vi "run.create_set_end.vi"(8 "error in":errorcluster, 10 "Time Stamp (Now)":timestamp format="%<%x %.3X>T", 11 "RunCreateStaging in":refnum<class "RunCreateStaging.lvclass">) -> (0 "error out":errorcluster, 3 "RunCreateStaging out":refnum<class "RunCreateStaging.lvclass">)   [LabVIEW 2020, in "RunCreateStaging.lvclass"]
doc: "Sets the end time for the run being created."
uses:
  RunCreateStaging.lvclass
  RunCreateStaging.lvclass/RunCreateStaging.ctl
  client.lvlib
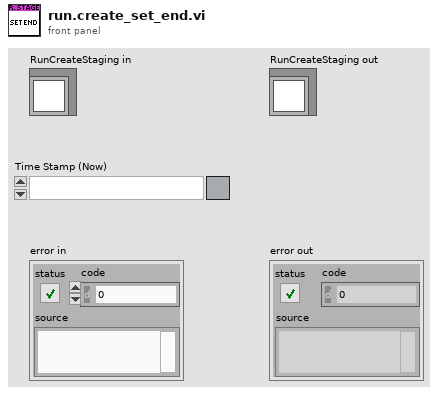
[diagram p1: front panel]
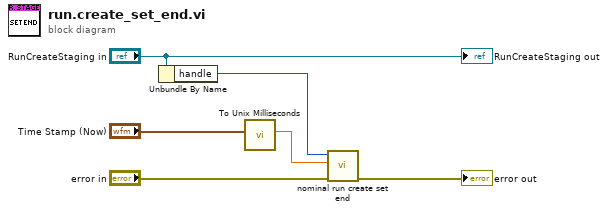
[diagram p0: block diagram]
diagram:
  n1 = Unbundle By Name("RunCreateStaging in") -> ("handle"=w4:i32)
  n2 = call "To Unix Milliseconds.vi"("Time Stamp (Now)"="Time Stamp (Now)") -> ("Unix Milliseconds"=w2:dbl)  [unwired: 10 in]
  n3 = call "nominal run create set end.vi"("error in (no error)"="error in", "end_ms"=w2, "staging"=w4) -> ("error out"=→"error out":errorcluster)  [unwired: 7 in, 1 out]
  "RunCreateStaging out" <- "RunCreateStaging in"
